vi "Create Events.vi"(8 "error in":errorcluster, 11 "Base Software in":refnum<class "Base Software.lvclass">) -> (0 "error out":errorcluster, 3 "Base Software out":refnum<class "Base Software.lvclass">)   [LabVIEW 2019, in "Base Software.lvlib" / "Main.lvlib" / "Base Software.lvclass"]
uses:
  Project/Base Software.lvclass
  C:/Users/Public/Documents/Development/builds/Engine/Engine.lvlibp/Project/Engine.lvclass
  builds/Engine/Engine.lvlibp/Custom Controls/System Status.ctl
  builds/Engine/Engine.lvlibp/Accessors/Write Fault Event.vi
  builds/Engine/Engine.lvlibp/Accessors/Write QuickStart Event.vi
  builds/Engine/Engine.lvlibp/Accessors/Write SafeBTE Event.vi
  builds/Engine/Engine.lvlibp/Accessors/Write TogglePower Event.vi
  builds/Engine/Engine.lvlibp/Accessors/Write SystemStatus Event.vi
  builds/Engine/Engine.lvlibp/Accessors/Write UUTSupply Event.vi
  builds/Engine/Engine.lvlibp/Accessors/Write UUT_Designator.vi
  builds/Engine/Engine.lvlibp/Accessors/Write Test_Operator.vi
  builds/Engine/Engine.lvlibp/Accessors/Write Test_Name.vi
  builds/Engine/Engine.lvlibp/Accessors/Write Test_Witness.vi
  builds/Engine/Engine.lvlibp/Accessors/Write Pedigree.vi
  builds/Engine/Engine.lvlibp/Accessors/Write Toggle Launch Event.vi
  builds/Engine/Engine.lvlibp/Accessors/Write Interface_Command Event.vi
  builds/Engine/Engine.lvlibp/Accessors/Write Telemetry_Descriptor.vi
  builds/Engine/Engine.lvlibp/Accessors/Write Asynch_Telemetry_Descriptor.vi
  builds/Engine/Engine.lvlibp/Accessors/Write Automation.vi
  builds/Engine/Engine.lvlibp/Project/Engine.lvclass
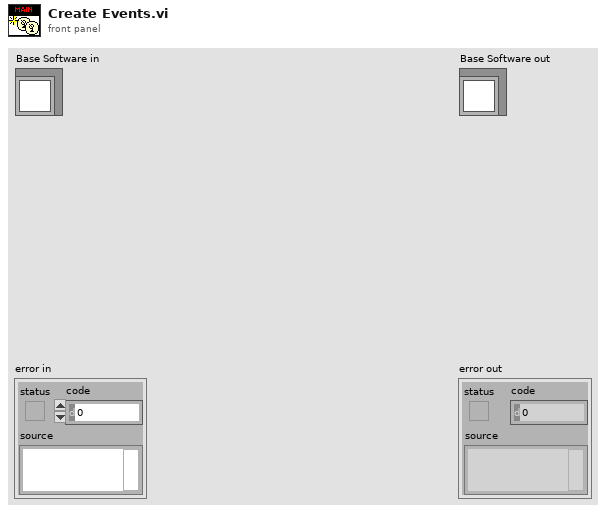
[diagram p1: front panel]
types:
  T1 = typedef "Engine.lvlibp/Engine.lvclass/System Status.ctl" = enum16{"Logged Off", "UUT_Info_Missing", "Idle", "Error", "Warning", "Loading", "Config", "Manual", "Automation", "Report_View", "Previous"}
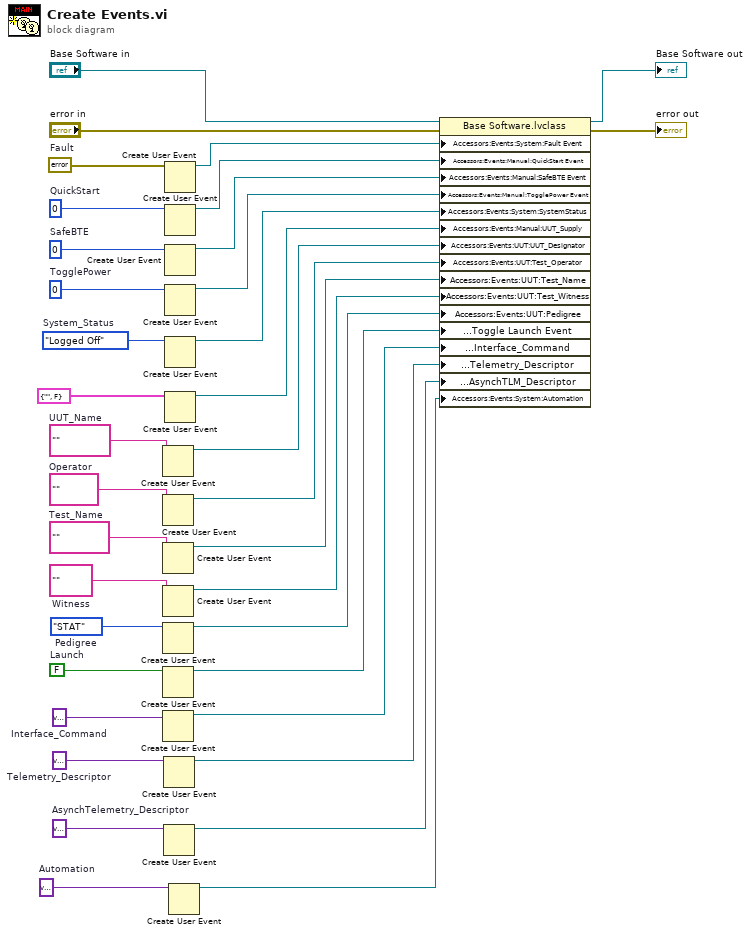
[diagram p0: block diagram]
diagram:
  w2 = variant  # Automation
  w3 = variant  # AsynchTelemetry_Descriptor
  w5 = variant  # Telemetry_Descriptor
  w8 = variant  # Interface_Command
  w10 = enum16{"STAT", "BB", "PT", "EM", "FT"}."STAT"  # Pedigree
  w11 = FALSE  # Launch
  w16 = ""  # Witness
  w17 = ""  # Test_Name
  w18 = ""  # Operator
  w20 = ""  # UUT_Name
  w27 = 0  # TogglePower
  w28 = System_Status."Logged Off"  # System_Status
  w30 = 0  # SafeBTE
  w31 = 0  # QuickStart
  w34 = errorcluster {"status"=FALSE, "code"=0, "source"=""}  # Fault
  n1 = Create User Event(user event datatype=w20) -> (user event=w19:refnum<user-event>)  [unwired: 1 in, 1 out]
  n2 = Create User Event(user event datatype=w18) -> (user event=w15:refnum<user-event>)  [unwired: 1 in, 1 out]
  n3 = Create User Event(user event datatype=w17) -> (user event=w14:refnum<user-event>)  [unwired: 1 in, 1 out]
  n4 = Create User Event(user event datatype=w16) -> (user event=w13:refnum<user-event>)  [unwired: 1 in, 1 out]
  n5 = Create User Event(user event datatype=w10) -> (user event=w9:refnum<user-event>)  [unwired: 1 in, 1 out]
  n6 = Create User Event(user event datatype=w11) -> (user event=w12:refnum<user-event>)  [unwired: 1 in, 1 out]
  n7 = Create User Event(user event datatype=w8) -> (user event=w7:refnum<user-event>)  [unwired: 1 in, 1 out]
  n8 = Create User Event(user event datatype=w5) -> (user event=w6:refnum<user-event>)  [unwired: 1 in, 1 out]
  n9 = Create User Event(user event datatype=w3) -> (user event=w4:refnum<user-event>)  [unwired: 1 in, 1 out]
  n10 = Create User Event(user event datatype=w34) -> (user event=w33:refnum<user-event>)  [unwired: 1 in, 1 out]
  n11 = Create User Event(user event datatype=w31) -> (user event=w32:refnum<user-event>)  [unwired: 1 in, 1 out]
  n12 = Create User Event(user event datatype=w30) -> (user event=w29:refnum<user-event>)  [unwired: 1 in, 1 out]
  n13 = Create User Event(user event datatype=w27) -> (user event=w26:refnum<user-event>)  [unwired: 1 in, 1 out]
  n14 = Create User Event(user event datatype=w28) -> (user event=w25:refnum<user-event>)  [unwired: 1 in, 1 out]
  n15 = Create User Event(user event datatype=cluster{"Supply":string, "Output":bool} {"Supply"="", "Output"=FALSE} ("event data")) -> (user event=w22:refnum<user-event>)  [unwired: 1 in, 1 out]
  n16 = Create User Event(user event datatype=w2) -> (user event=w1:refnum<user-event>)  [unwired: 1 in, 1 out]
  n17 = property class="Base Software.lvclass"(reference="Base Software in", error in="error in", "Accessors:Events:System:Fault Event"=w33, "Accessors:Events:Manual:QuickStart Event"=w32, "Accessors:Events:Manual:SafeBTE Event"=w29, "Accessors:Events:Manual:TogglePower Event"=w26, "Accessors:Events:System:SystemStatus"=w25, "Accessors:Events:Manual:UUT_Supply"=w22, "Accessors:Events:UUT:UUT_Designator"=w19, "Accessors:Events:UUT:Test_Operator"=w15, "Accessors:Events:UUT:Test_Name"=w14, "Accessors:Events:UUT:Test_Witness"=w13, "Accessors:Events:UUT:Pedigree"=w9, "Accessors:Events:Manual:Toggle Launch Event"=w12, "Accessors:Events:Interface:Interface_Command"=w7, "Accessors:Events:Interface:Telemetry_Descriptor"=w6, "Accessors:Events:Interface:AsynchTLM_Descriptor"=w4, "Accessors:Events:System:Automation"=w1) -> (reference out=→"Base Software out":refnum<class "Base Software.lvclass">, error out=→"error out":errorcluster)
